vi "Session Information.vi"(7 "Section Name":string, 8 "error in (no error)":errorcluster, 11 "Config in":refnum<class "LabVIEW-Config.lvclass">) -> (0 "error out":errorcluster, 2 "Session Information":T1, 3 "Config out":refnum<class "LabVIEW-Config.lvclass">)   [LabVIEW 2017, in "LabVIEW-Config.lvlib" / "LabVIEW-Config.lvclass"]
uses:
  LabVIEW-Config.lvclass
  SessionInfo.ctl
  LabVIEW-Config.lvclass/LabVIEW-Config.ctl
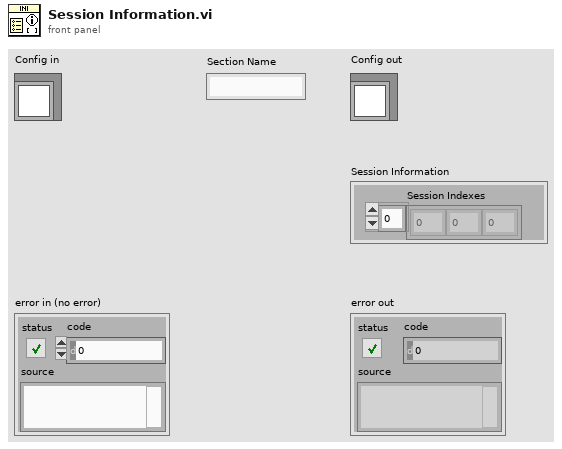
[diagram p1: front panel]
types:
  T1 = typedef "LabVIEW-Config.lvlib/LabVIEW-Config.lvclass/SessionInfo.ctl" = cluster{"Session Indexes":i32[]}
  T2 = typedef "LabVIEW-Config.lvlib/LabVIEW-Config.lvclass/LineToken.ctl" = enum8{"comment", "section", "key", "more"}
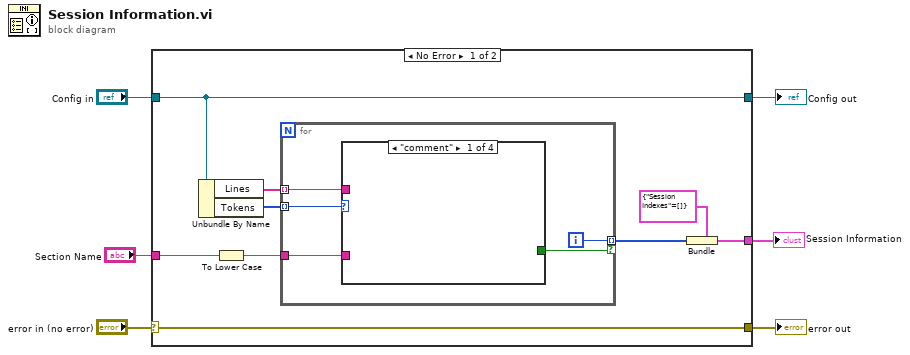
[diagram p0: block diagram]
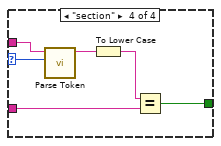
[diagram p4: hidden frame]
diagram:
  n1 = case shown="No Error" "error in (no error)" {
    selector: "error in (no error)" -> [w13 w28]
    tunnel: "Config in" -> [w11 w27]
    tunnel: [w13 w28] -> w5
    tunnel: [w11 w27] -> w3
    tunnel: "Section Name" -> [w7 _]
    tunnel: [w9 _] -> w1
    frame No Error {
      n2 = Unbundle By Name(w11) -> ("Lines"=w14:string[], "Tokens"=w15:T2[])
      n3 = To Lower Case(string=w7) -> (all lower case string=w12:string)
      n4 = for {
        tunnel: w15 -> [w20] mode=indexing
        tunnel: w14 -> [w19] mode=indexing
        tunnel: w12 -> [w18]
        tunnel: [w17] -> w10 mode=indexing if=w16
        i -> [w17]
        n5 = case shown="\"comment\"" w20 {
          selector: w20 -> [_ _ _ w23]
          tunnel: w19 -> [_ _ _ w24]
          tunnel: w18 -> [_ _ _ w26]
          tunnel: [_ _ _ w21] -> w16
          frame "comment" {
          }
          frame "more" {
          }
          frame "key" {
          }
          frame "section" {
            n6 = call "Parse Token.vi"("Token"=w23, "Line"=w24) -> ("Name"=w22:string)  [unwired: 8 in, 1 out]
            n7 = To Lower Case(string=w22) -> (all lower case string=w25:string)
            n8 = Equal?(x=w25, y=w26) -> (x = y?=w21:bool)
          }
        }
      }
      n9 = Bundle(cluster=T1 {"Session Indexes"=[]}, "Session Indexes"=w10) -> (w9:T1)
    }
    frame Error {
    }
  }
  "error out" <- w5
  "Config out" <- w3
  "Session Information" <- w1
